vi "BoxAngleComp.vi"(11 "Raw":cluster{dbl, dbl, dbl}) -> (3 "Compensated":cluster{dbl, dbl, dbl})   [LabVIEW 2019]
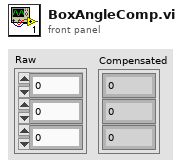
[diagram p1: front panel]
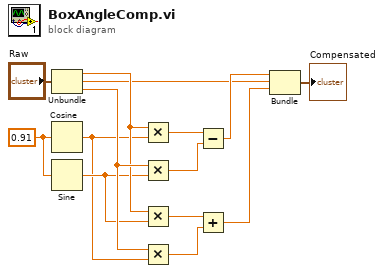
[diagram p0: block diagram]
diagram:
  w14 = 0.91 ("x")
  n1 = Unbundle("Raw") -> (w5:dbl, w3:dbl, w9:dbl)
  n2 = Cosine(x=w14) -> (cos(x)=w1:dbl)
  n3 = Sine(x=w14) -> (sin(x)=w2:dbl)
  n4 = Multiply(x=w5, y=w1) -> (x*y=w13:dbl)
  n5 = Multiply(x=w9, y=w2) -> (x*y=w12:dbl)
  n6 = Multiply(x=w5, y=w2) -> (x*y=w11:dbl)
  n7 = Multiply(x=w9, y=w1) -> (x*y=w10:dbl)
  n8 = Subtract(x=w13, y=w12) -> (x-y=w4:dbl)
  n9 = Add(x=w11, y=w10) -> (x+y=w7:dbl)
  n10 = Bundle(w4, w3, w7) -> (→"Compensated":cluster{dbl, dbl, dbl})  [unwired: 1 in]
